vi "State Actor Teardown.vi"(7 "Self Actor":refnum<class "Self Actor.lvclass">, 10 "Error":errorcluster, 11 "Msging Self Actor State in":refnum<class "Msging Self Actor State.lvclass">) -> (0 "error out":errorcluster, 2 "Teardown?":bool)   [LabVIEW 2021, in "LVCAM.lvlib" / "Msging Self Actor State.lvclass"]
uses:
  Msging Self Actor State.lvclass
  Self Actor/Self Actor.lvclass
  C:/PPLs/LabVIEW-Composed-Actor-Model-LVCAM/LabVIEW-Composed-Actor-Model-LVCAM/LVCAM/LVCAM/Actor/Actor.lvclass
  Msgs/Actor Destroy/Actor Destroy Msg Strategy/Actor Destroy Msg Strategy.lvclass
  C:/PPLs/LabVIEW-Composed-Actor-Model-LVCAM/LabVIEW-Composed-Actor-Model-LVCAM/LVCAM/LVCAM/Msg Strategy/Msg Strategy.lvclass
  Msging Self Actor State.lvclass/Msging Self Actor State.ctl
  Self Actor/Self Msg Send.vi
  C:/PPLs/LabVIEW-Composed-Actor-Model-LVCAM/LabVIEW-Composed-Actor-Model-LVCAM/LVCAM/Msgs/Actor Create/Actor Create/Actor Create.lvclass
  C:/PPLs/LabVIEW-Composed-Actor-Model-LVCAM/LabVIEW-Composed-Actor-Model-LVCAM/LVCAM/Msgs/Actor Destroy/Actor Destroy/Actor Destroy.lvclass
  C:/PPLs/LabVIEW-Composed-Actor-Model-LVCAM/LabVIEW-Composed-Actor-Model-LVCAM/LVCAM/Msgs/Actor Last Ack/Actor Last Ack/Actor Last Ack.lvclass
  C:/PPLs/LabVIEW-Composed-Actor-Model-LVCAM/LabVIEW-Composed-Actor-Model-LVCAM/LVCAM/LVCAM/Self Actor/Self Actor.lvclass
  C:/PPLs/LabVIEW-Composed-Actor-Model-LVCAM/LabVIEW-Composed-Actor-Model-LVCAM/LVCAM/Msgs/Actor Destroy/Actor Destroy Msg Strategy/Actor Destroy Msg Strategy.lvclass
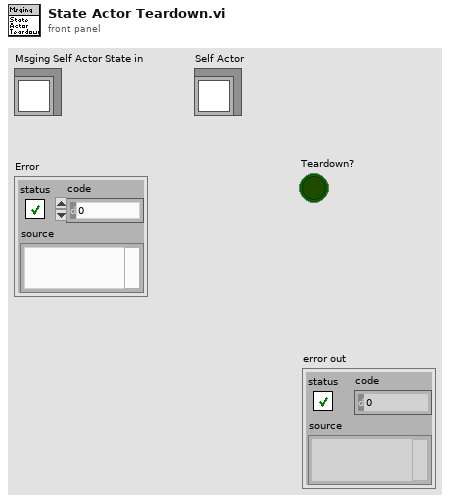
[diagram p1: front panel]
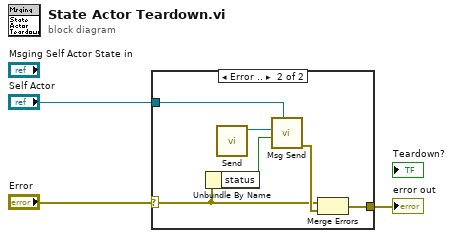
[diagram p0: block diagram]
diagram:
  n1 = case shown="Error .." "Error" {
    selector: "Error" -> [_ w5]
    tunnel: [_ w7] -> w1
    tunnel: "Self Actor" -> [_ w8]
    frame No Error {
    }
    frame Error {
      n2 = Unbundle By Name(w5) -> ("status"=w4:bool)
      n3 = call "Send.vi"() -> ("Actor Destroy Msg Strategy out"=w9:refnum<class "Actor Destroy Msg Strategy.lvclass">)  [unwired: 11 in]
      n4 = call-poly "Msg Send.vi"("Actor"=w8, "Priority Msg?"=w4, "Msg"=w9) -> ("error out"=w6:errorcluster)  [unwired: 8 in]
      n5 = Merge Errors(w5, w6) -> (w7:errorcluster)
    }
  }
  "error out" <- w1
